vi "GDSFile_RecursiveFileList.vi"(4 "Folders to Exclude":string[](array[string]), 6 "pattern":string, 7 "StopWhenNoOfFilesFound":i32, 8 "error in (no error)":errorcluster, 9 "Continue Recursing on Error? (F)":bool, 10 "Treat LLBs as Folders?":bool, 11 "Folder Path":path) -> (0 "error out":errorcluster, 1 "Number of Files":i32, 2 "All Files in Dir":path[](array[path]), 3 "dup Folder Path":path, 5 "All Folders":path[](array[path]))   [LabVIEW 2014]
doc: "Lists the contents of a folder or LLB. In order for this VI to work correctly, the LLB must have a .llb file extension."
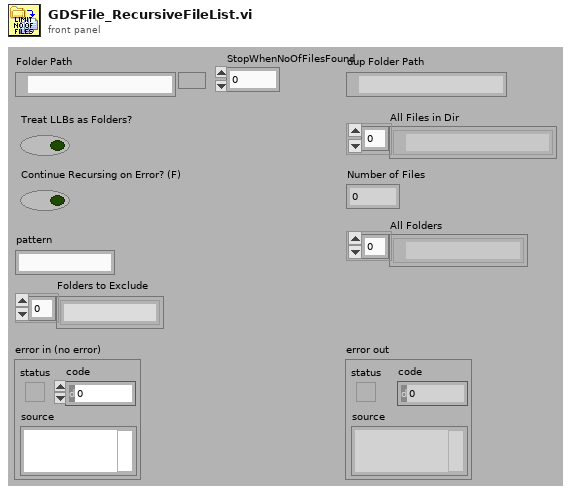
[diagram p1: front panel]
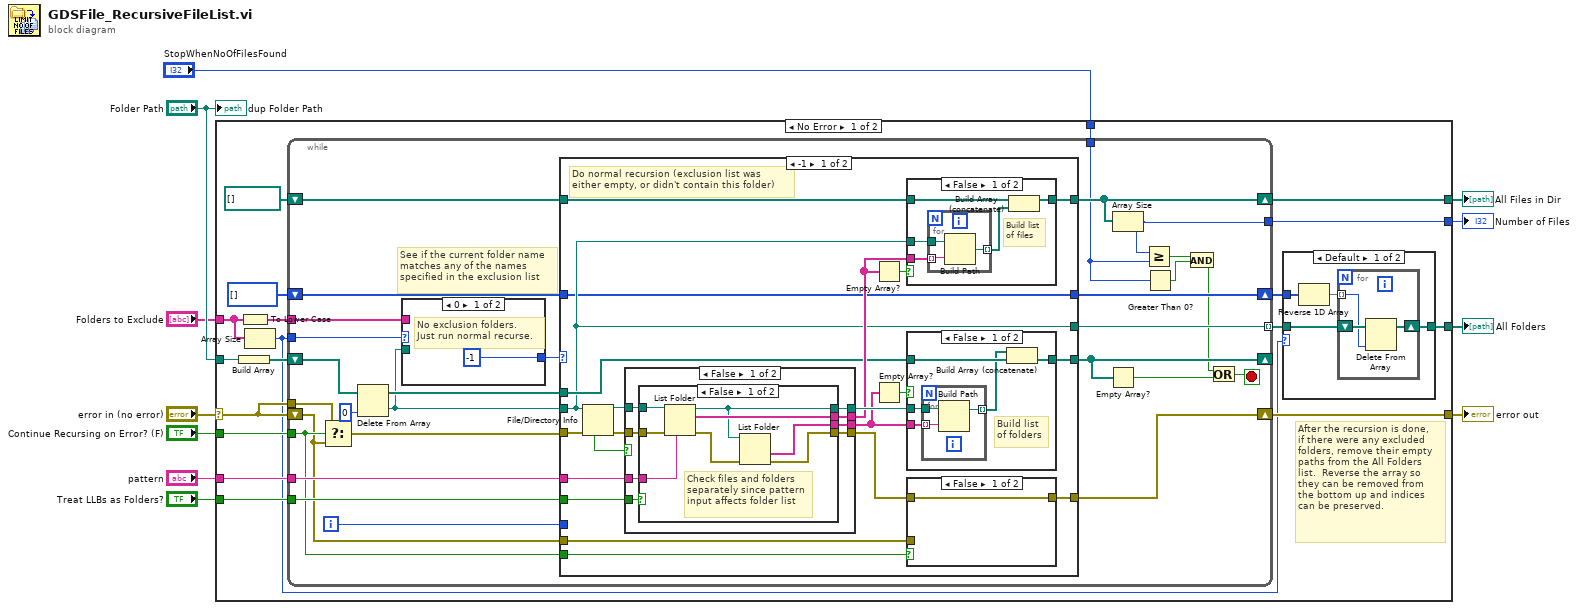
[diagram p0: block diagram]
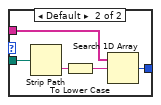
[diagram p3: hidden frame]
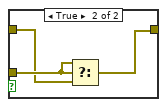
[diagram p5: hidden frame]
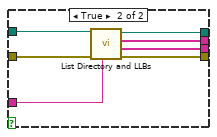
[diagram p6: hidden frame]
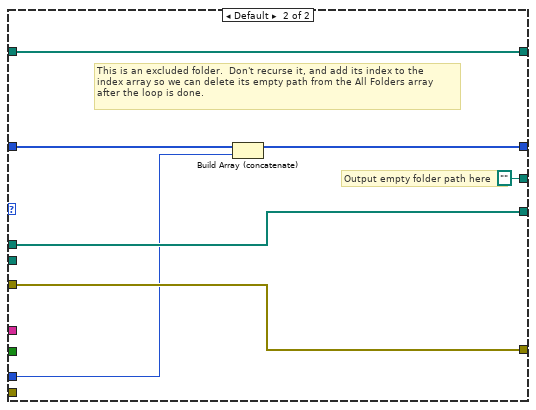
[diagram p9: hidden frame]
diagram:
  n1 = case shown="No Error" "error in (no error)" {
    selector: "error in (no error)" -> [w21 w147]
    tunnel: "Folder Path" -> [w29 _]
    tunnel: [w23 _] -> w11
    tunnel: [w13 _] -> w10
    tunnel: [w24 w147] -> w9
    tunnel: "Treat LLBs as Folders?" -> [w26 _]
    tunnel: [w15 _] -> w6
    tunnel: "pattern" -> [w25 _]
    tunnel: "Continue Recursing on Error? (F)" -> [w22 _]
    tunnel: "Folders to Exclude" -> [w18 _]
    tunnel: "StopWhenNoOfFilesFound" -> [w12 _]
    frame No Error {
      # "After the recursion is done,\nif there were any excluded\nfolders, remove their empty\npaths from the All Folders\nlist.  Reverse the array so\nthey can be removed from\nthe bottom up and indices\ncan be preserved."
      n2 = Build Array(w29) -> (w28:path[])
      n3 = To Lower Case(string=w18) -> (all lower case string=w20:string[])
      n4 = Array Size(array=w18) -> (size(s)=w16:i32)
      n5 = while {
        shift-left: path[] [] ("Array Constant") -> [w64]
        shift-right: [w45] -> w23
        shift-left: w28 -> [w65]
        shift-right: [w61] -> _
        shift-right: [w56] -> w24
        shift-left: w21 -> [w55]
        tunnel: w26 -> [w63]
        tunnel: [w52] -> w17 mode=indexing
        tunnel: w25 -> [w62]
        tunnel: w22 -> [w57]
        tunnel: w21 -> [w58]
        tunnel: w20 -> [w48]
        shift-right: [w51] -> w14
        shift-left: i32[] [] -> [w53]
        tunnel: w16 -> [w49]
        tunnel: [w42] -> w13
        tunnel: w12 -> [w40]
        i -> [w50]
        stop <- w43 stop-if-true
        # "See if the current folder name\nmatches any of the names\nspecified in the exclusion list"
        n6 = Select(t=w58, s=w57, f=w55) -> (s? t:f=w59:errorcluster)
        n7 = Delete From Array(array=w65, index=0) -> (deleted portion=w47:path, array with subset deleted=w54:path[])  [unwired: 1 in]
        n8 = case shown="0" w49 {
          tunnel: w48 -> [_ w68]
          tunnel: w47 -> [_ w71]
          tunnel: [-1 ("index of element") w67] -> w46
          frame 0 {
            # "No exclusion folders.\nJust run normal recurse."
          }
          frame Default {
            n9 = Strip Path(path=w71) -> (name=w70:string)  [unwired: 1 out]
            n10 = To Lower Case(string=w70) -> (all lower case string=w69:string)
            n11 = Search 1D Array(1D array=w68, element=w69) -> (index of element=w67:i32)  [unwired: 1 out]
          }
        }
        n12 = case shown="-1" w46 {
          tunnel: [w92 w146] -> w45
          tunnel: w64 -> [w91 w146]
          tunnel: w63 -> [w89 _]
          tunnel: w62 -> [w88 _]
          tunnel: [w85 w145] -> w61
          tunnel: w47 -> [w73 _]
          tunnel: w59 -> [w81 w144]
          tunnel: w57 -> [w79 _]
          tunnel: [w78 w144] -> w56
          tunnel: w55 -> [w77 _]
          tunnel: w54 -> [w74 w145]
          tunnel: w53 -> [w72 w143]
          tunnel: [w73 path ""] -> w52
          tunnel: [w72 w142] -> w51
          tunnel: w50 -> [_ w141]
          frame -1 {
            # "Do normal recursion (exclusion list was\neither empty, or didn't contain this folder)"
            n13 = File/Directory Info(path=w73, error in=w81) -> (path out=w83:path, error out=w84:errorcluster, shortcut=w82:bool)  [unwired: 4 out]
            n14 = case shown="False" w82 {
              tunnel: [w113 _] -> w75
              tunnel: [w112 w130] -> w90
              tunnel: [w111 w129] -> w80
              tunnel: w89 -> [w110 _]
              tunnel: w88 -> [w109 _]
              tunnel: [w108 _] -> w87
              tunnel: w84 -> [w107 w129]
              tunnel: w83 -> [w106 w130]
              frame False {
                n15 = case shown="False" w110 {
                  tunnel: [w121 w125] -> w113
                  tunnel: [w115 w124] -> w108
                  tunnel: w106 -> [w120 w128]
                  tunnel: [w114 w126] -> w112
                  tunnel: [w116 w123] -> w111
                  tunnel: w107 -> [w119 w127]
                  tunnel: w109 -> [w118 w122]
                  frame False {
                    # "Check files and folders\nseparately since pattern\ninput affects folder list"
                    n16 = List Folder(path=w120, pattern=w118, error in=w119) -> (path out=w114:path, filenames=w121:string[], error out=w117:errorcluster)  [unwired: 2 out]
                    n17 = List Folder(path=w114, error in=w117) -> (folder names=w115:string[], error out=w116:errorcluster)  [unwired: 4 out]
                  }
                  frame True {
                    n18 = call <vilib>:"List Directory and LLBs.vi"("pattern"=w122, "error in (no error)"=w127, "Folder Path"=w128) -> ("error out"=w123:errorcluster, "Folders and LLBs"=w124:string[], "Files sans LLBs"=w125:string[], "dup Folder Path"=w126:path)  [unwired: 5 out]
                  }
                }
              }
              frame True {
                # "Do not attempt to recurse the contents\nof folder shortcuts"
              }
            }
            n19 = Empty Array?(array=w75) -> (empty?=w76:bool)
            n20 = Empty Array?(array=w87) -> (empty?=w86:bool)
            n21 = case shown="False" w76 {
              tunnel: [w97 w101] -> w92
              tunnel: w75 -> [w96 _]
              tunnel: w91 -> [w95 w101]
              tunnel: w73 -> [w93 _]
              frame False {
                # "Build list of files"
                n22 = for {
                  tunnel: w96 -> [w99] mode=indexing
                  tunnel: w93 -> [w100]
                  tunnel: [w98] -> w94 mode=indexing
                  n23 = Build Path(base path=w100, name or relative path=w99) -> (appended path=w98:path)
                }
                n24 = Build Array (concatenate)(w95, w94) -> (w97:path[])
              }
              frame True {
              }
            }
            n25 = case shown="False" w86 {
              tunnel: w74 -> [w133 w139]
              tunnel: [w134 w139] -> w85
              tunnel: w90 -> [w135 _]
              tunnel: w87 -> [w131 _]
              frame False {
                # "Build list\nof folders"
                n26 = for {
                  tunnel: w135 -> [w138]
                  tunnel: [w137] -> w132 mode=indexing
                  tunnel: w131 -> [w136] mode=indexing
                  n27 = Build Path(base path=w138, name or relative path=w136) -> (appended path=w137:path)
                }
                n28 = Build Array (concatenate)(w132, w133) -> (w134:path[])
              }
              frame True {
              }
            }
            n29 = case shown="False" w79 {
              tunnel: w80 -> [w102 w104]
              tunnel: [w102 w103] -> w78
              tunnel: w77 -> [_ w105]
              frame False {
              }
              frame True {
                n30 = Select(t=w105, s=w105, f=w104) -> (s? t:f=w103:errorcluster)
              }
            }
          }
          frame Default {
            # "Output empty folder path here"
            # "This is an excluded folder.  Don't recurse it, and add its index to the\nindex array so we can delete its empty path from the All Folders array\nafter the loop is done."
            n31 = Build Array (concatenate)(w143, w141) -> (w142:i32[])
          }
        }
        n32 = Empty Array?(array=w61) -> (empty?=w44:bool)
        n33 = Array Size(array=w45) -> (size(s)=w42:i32)
        n34 = Greater Or Equal?(x=w42, y=w40) -> (x >= y?=w41:bool)
        n35 = Greater Than 0?(x=w40) -> (x > 0?=w39:bool)
        n36 = And(x=w41, y=w39) -> (x .and. y?=w38:bool)
        n37 = Or(x=w38, y=w44) -> (x .or. y?=w43:bool)
      }
      n38 = case shown="Default" w16 {
        tunnel: w17 -> [w32 w37]
        tunnel: [w31 w37] -> w15
        tunnel: w14 -> [w33 _]
        frame Default {
          n39 = Reverse 1D Array(array=w33) -> (reversed array=w30:i32[])
          n40 = for {
            shift-right: [w35] -> w31
            shift-left: w32 -> [w36]
            tunnel: w30 -> [w34] mode=indexing
            n41 = Delete From Array(array=w36, index=w34) -> (array with subset deleted=w35:path[])  [unwired: 1 in, 1 out]
          }
        }
        frame 0 {
          # "No excluded folders.\nDon't run the code that\ndeletes excluded folder\nindices."
        }
      }
    }
    frame Error {
    }
  }
  "All Files in Dir" <- w11
  "Number of Files" <- w10
  "error out" <- w9
  "All Folders" <- w6
  "dup Folder Path" <- "Folder Path"
